vi "View_2FITScomp.vi"() -> ()   [LabVIEW 2020]
panel:
  in  "stop":bool
  out "Slice":sgl[][](graph)
  out "Image":sgl[][](graph)
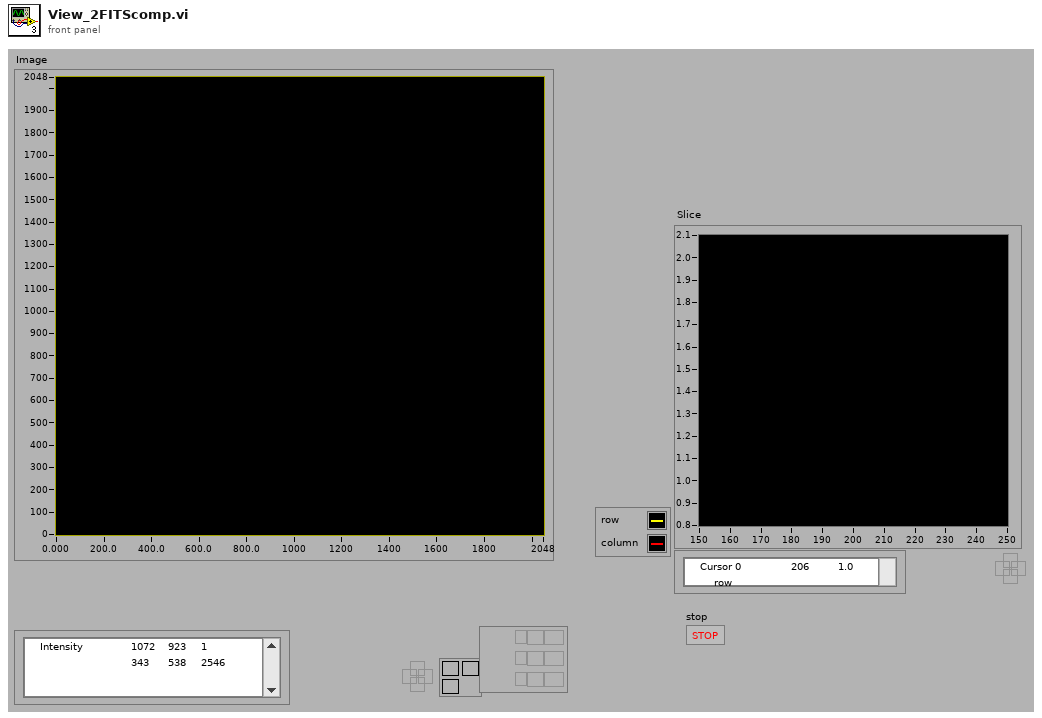
[diagram p1: front panel]
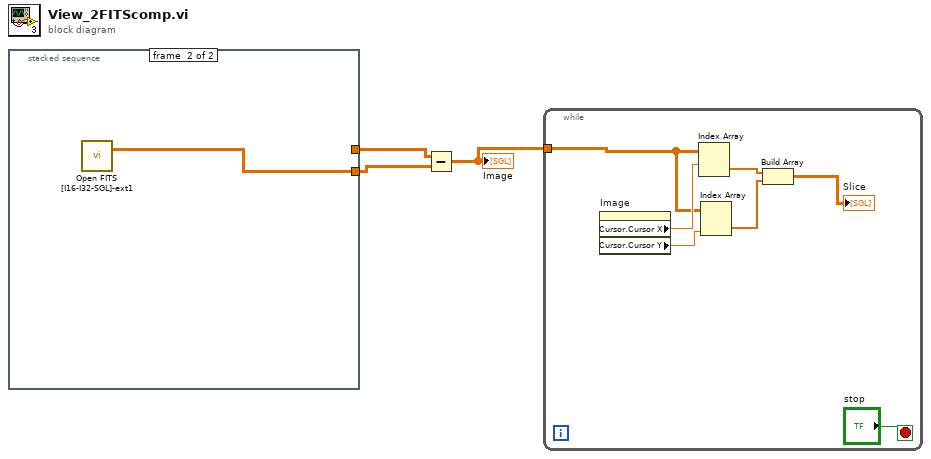
[diagram p0: block diagram]
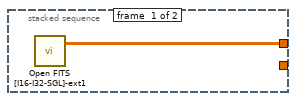
[diagram p2: hidden frame]
diagram:
  n1 = stacked-sequence {
    tunnel: [w4 _] -> w3
    tunnel: [_ w5] -> w2
    frame #0 {
      n2 = call "Open FITS [I16-I32-SGL]-ext1.vi"() -> ("Image"=w4:sgl[][])  [unwired: 12 in, 3 out]
    }
    frame #1 {
      n3 = call "Open FITS [I16-I32-SGL]-ext1.vi"() -> ("Image"=w5:sgl[][])  [unwired: 12 in, 3 out]
    }
  }
  n4 = Subtract(x=w3, y=w2) -> (x-y=w1:sgl[][])
  "Image" <- w1
  n5 = while {
    tunnel: w1 -> [w9]
    stop <- "stop" stop-if-true
    n6 = property on="Image" class="IntGraph (strict)"() -> ("Cursor.Cursor X"=w12:dbl, "Cursor.Cursor Y"=w11:dbl)  [unwired: 2 in, 2 out]
    n7 = Index Array(array=w9, index (row)=w12) -> (element=w10:sgl[])  [unwired: 1 in]
    n8 = Index Array(array=w9, index (col)=w11) -> (element=w8:sgl[])  [unwired: 1 in]
    n9 = Build Array(w10, w8) -> (→"Slice":sgl[][])
  }
